vi "Update Build Specs and Build.vi"(8 "error in":errorcluster, 9 "CD lvproj name":string, 10 "CD name":string, 11 "custom device path":path) -> (0 "error out":errorcluster, 3 "custom device path out":path)   [LabVIEW 2020, in "Template Tool.lvlib"]
uses:
  Template Tool.lvlib
  <vilib>/AppBuilder/AB_API/SDIST/NI_AB_API_SDIST.lvclass
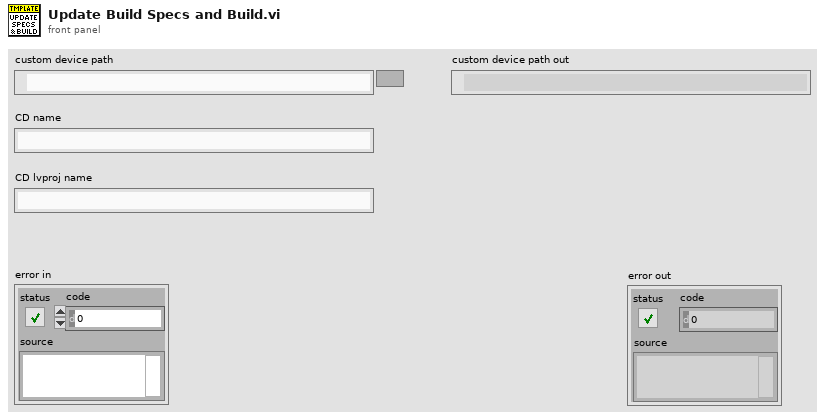
[diagram p1: front panel]
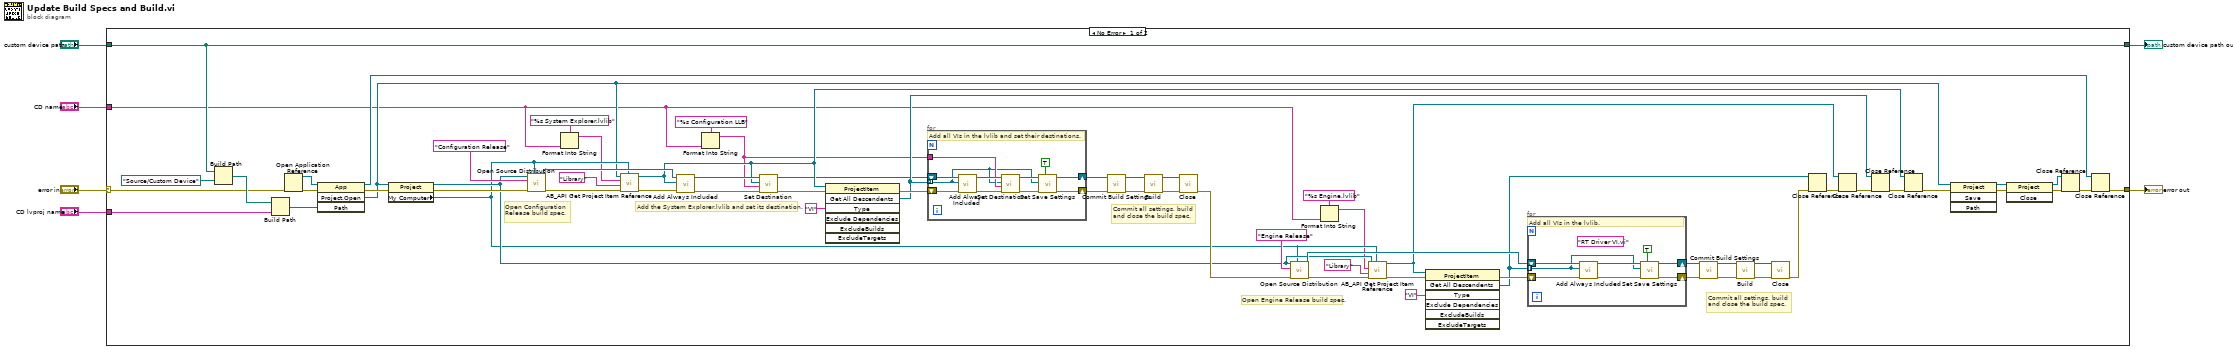
[diagram p0: block diagram]
diagram:
  n1 = case shown="No Error" "error in" {
    selector: "error in" -> [w71 w94]
    tunnel: "custom device path" -> [w55 w93]
    tunnel: [w57 w94] -> w6
    tunnel: [w55 w93] -> w3
    tunnel: "CD lvproj name" -> [w19 _]
    tunnel: "CD name" -> [w18 _]
    frame No Error {
      # "Commit all settings, build and close the build spec."
      # "Open Engine Release build spec."
      # "Commit all settings, build and close the build spec."
      # "Add the System Explorer.lvlib and set its destination."
      # "Open Configuration Release build spec."
      n2 = Build Path(base path=w55, name or relative path=path "Source/Custom Device") -> (appended path=w72:path)
      n3 = Build Path(base path=w72, name or relative path=w19) -> (appended path=w68:path)
      n4 = Open Application Reference(8:w71) -> (0:w70:errorcluster, 3:w69:refnum<vi>)  [unwired: 3 in]
      n5 = invoke class="App" method="Project.Open"(reference=w69, error in=w70, "Path"=w68) -> (reference out=w51:refnum<vi>, error out=w67:errorcluster, "Project:Open"=w22:refnum<vi>)  [unwired: 1 in, 1 out]
      n6 = property class="Project"(reference=w22, error in=w67) -> (reference out=w36:refnum<vi>, error out=w62:errorcluster, "My Computer"=w35:refnum<vi>)
      n7 = call <vilib>:"Open Source Distribution.vi"("TargetItem Refnum"=w35, "error in (no error)"=w62, "Build specification name"="Configuration Release", "Project Refnum"=w36) -> ("error out"=w64:errorcluster, "SDIST out"=w60:refnum<class "NI_AB_API_SDIST.lvclass">)  [unwired: 6 in]
      n8 = Format Into String(format string="%s System Explorer.lvlib" ("Build specification name"), w18) -> (resulting string=w27:string)  [unwired: 2 in, 1 out]
      n9 = call <vilib>:"AB_API Get Project Item Reference.vi"("TargetItem Refnum"=w35, "error in (no error)"=w64, "Type"="Library", "Name"=w27, "Project Refnum"=w22) -> ("error out"=w56:errorcluster, "ProjectItem Refnum"=w45:refnum<vi>)  [unwired: 4 in, 1 out]
      n10 = call-dynamic "Add Always Included.vi"("error in (no error)"=w56, "ProjectItem Refnum"=w45, "SDIST in"=w60) -> ("error out"=w47:errorcluster, "SDIST out"=w48:refnum<class "NI_AB_API_SDIST.lvclass">)  [unwired: 7 in]
      n11 = Format Into String(format string="%s Configuration LLB" ("Destination label"), w18) -> (resulting string=w29:string)  [unwired: 2 in, 1 out]
      n12 = call-dynamic "Set Destination.vi"("error in (no error)"=w47, "Destination label"=w29, "ProjectItem Refnum"=w45, "SDIST in"=w48) -> ("error out"=w46:errorcluster, "SDIST out"=w30:refnum<class "NI_AB_API_SDIST.lvclass">)  [unwired: 6 in]
      n13 = invoke class="ProjectItem" method="Get All Descendents"(reference=w45, error in=w46, "Type"="VI") -> (error out=w52:errorcluster, "All Descendents"=w49:refnum<vi>[])  [unwired: 4 in, 5 out]
      n14 = for {
        shift-right: [w83] -> w53
        shift-left: w30 -> [w92]
        shift-right: [w85] -> w54
        shift-left: w52 -> [w91]
        tunnel: w49 -> [w82] mode=indexing
        tunnel: w29 -> [w88]
        # "Add all VIs in the lvlib and set their destinations."
        n15 = call-dynamic "Add Always Included.vi"("error in (no error)"=w91, "ProjectItem Refnum"=w82, "SDIST in"=w92) -> ("error out"=w89:errorcluster, "SDIST out"=w90:refnum<class "NI_AB_API_SDIST.lvclass">)  [unwired: 7 in]
        n16 = call-dynamic "Set Destination.vi"("error in (no error)"=w89, "Destination label"=w88, "ProjectItem Refnum"=w82, "SDIST in"=w90) -> ("error out"=w86:errorcluster, "SDIST out"=w84:refnum<class "NI_AB_API_SDIST.lvclass">)  [unwired: 6 in]
        n17 = call-dynamic "Set Save Settings.vi"("Remove block diagram (false)"=TRUE, "error in (no error)"=w86, "ProjectItem Refnum"=w82, "SDIST in"=w84) -> ("error out"=w85:errorcluster, "SDIST out"=w83:refnum<class "NI_AB_API_SDIST.lvclass">)  [unwired: 6 in]
      }
      n18 = call-dynamic "Commit Build Settings.vi"("error in (no error)"=w54, "SDIST in"=w53) -> ("error out"=w15:errorcluster, "SDIST out"=w17:refnum<class "NI_AB_API_SDIST.lvclass">)  [unwired: 8 in]
      n19 = call-dynamic "Build.vi"("error in (no error)"=w15, "SDIST in"=w17) -> ("error out"=w14:errorcluster, "SDIST out"=w16:refnum<class "NI_AB_API_SDIST.lvclass">)  [unwired: 6 in, 2 out]
      n20 = call-dynamic "Close.vi"("error in (no error)"=w14, "SDIST in"=w16) -> ("error out"=w41:errorcluster)  [unwired: 9 in]
      n21 = call <vilib>:"Open Source Distribution.vi"("TargetItem Refnum"=w35, "error in (no error)"=w41, "Build specification name"="Engine Release", "Project Refnum"=w36) -> ("error out"=w43:errorcluster, "SDIST out"=w37:refnum<class "NI_AB_API_SDIST.lvclass">)  [unwired: 6 in]
      n22 = Format Into String(format string="%s Engine.lvlib" ("Build specification name"), w18) -> (resulting string=w25:string)  [unwired: 2 in, 1 out]
      n23 = call <vilib>:"AB_API Get Project Item Reference.vi"("TargetItem Refnum"=w35, "error in (no error)"=w43, "Type"="Library", "Name"=w25, "Project Refnum"=w36) -> ("error out"=w38:errorcluster, "ProjectItem Refnum"=w31:refnum<vi>)  [unwired: 4 in, 1 out]
      n24 = invoke class="ProjectItem" method="Get All Descendents"(reference=w31, error in=w38, "Type"="VI") -> (error out=w40:errorcluster, "All Descendents"=w32:refnum<vi>[])  [unwired: 4 in, 5 out]
      n25 = for {
        shift-right: [w78] -> w7
        shift-left: w37 -> [w81]
        shift-right: [w76] -> w8
        shift-left: w40 -> [w80]
        tunnel: w32 -> [w75] mode=indexing
        (unwired) "RT Driver VI.vi" ("Build specification name")
        # "Add all VIs in the lvlib."
        n26 = call-dynamic "Add Always Included.vi"("error in (no error)"=w80, "ProjectItem Refnum"=w75, "SDIST in"=w81) -> ("error out"=w77:errorcluster, "SDIST out"=w79:refnum<class "NI_AB_API_SDIST.lvclass">)  [unwired: 7 in]
        n27 = call-dynamic "Set Save Settings.vi"("Remove block diagram (false)"=TRUE, "error in (no error)"=w77, "ProjectItem Refnum"=w75, "SDIST in"=w79) -> ("error out"=w76:errorcluster, "SDIST out"=w78:refnum<class "NI_AB_API_SDIST.lvclass">)  [unwired: 6 in]
      }
      n28 = call-dynamic "Commit Build Settings.vi"("error in (no error)"=w8, "SDIST in"=w7) -> ("error out"=w12:errorcluster, "SDIST out"=w10:refnum<class "NI_AB_API_SDIST.lvclass">)  [unwired: 8 in]
      n29 = call-dynamic "Build.vi"("error in (no error)"=w12, "SDIST in"=w10) -> ("error out"=w13:errorcluster, "SDIST out"=w11:refnum<class "NI_AB_API_SDIST.lvclass">)  [unwired: 6 in, 2 out]
      n30 = call-dynamic "Close.vi"("error in (no error)"=w13, "SDIST in"=w11) -> ("error out"=w9:errorcluster)  [unwired: 9 in]
      n31 = Close Reference(reference=w32, error in (no error)=w9) -> (error out=w34:errorcluster)
      n32 = Close Reference(reference=w31, error in (no error)=w34) -> (error out=w33:errorcluster)
      n33 = Close Reference(reference=w49, error in (no error)=w33) -> (error out=w50:errorcluster)
      n34 = Close Reference(reference=w45, error in (no error)=w50) -> (error out=w23:errorcluster)
      n35 = invoke class="Project" method="Save"(reference=w22, error in=w23) -> (reference out=w21:refnum<vi>, error out=w20:errorcluster)  [unwired: 2 in, 2 out]
      n36 = invoke class="Project" method="Close"(reference=w21, error in=w20) -> (reference out=w58:refnum<vi>, error out=w59:errorcluster)  [unwired: 1 in, 1 out]
      n37 = Close Reference(reference=w58, error in (no error)=w59) -> (error out=w65:errorcluster)
      n38 = Close Reference(reference=w51, error in (no error)=w65) -> (error out=w57:errorcluster)
    }
    frame Error {
    }
  }
  "error out" <- w6
  "custom device path out" <- w3
